vi "PQ_asynchron_sample.vi"() -> ()   [LabVIEW 2019, in "libpqutility64.lvlib"]
doc: "example to show how to communicate asyncronous wir PostgreSQL"
uses:
  libpqutility64.lvlib
  libpqlv64/src/PQgetvalue.vi
  libpqlv64/src/PQnfields.vi
  libpqlv/libpqlv.lvlib
panel:
  out "parameterstatus":string
  out "PQbinaryTuples":i32
  out "PQprotocolVersion":u32
  out "PQnTuples":i32
  out "PQsendQuery":i32
  out "PQerrorMessage":string
  out "PQresultErrorMessage":string
  in  "query":string
  out "PQresultStatus":T1(ring)
  out "PQStatus":T2(ring)
  out "Tabelle":string[][](table)
  in  "conninfo":string
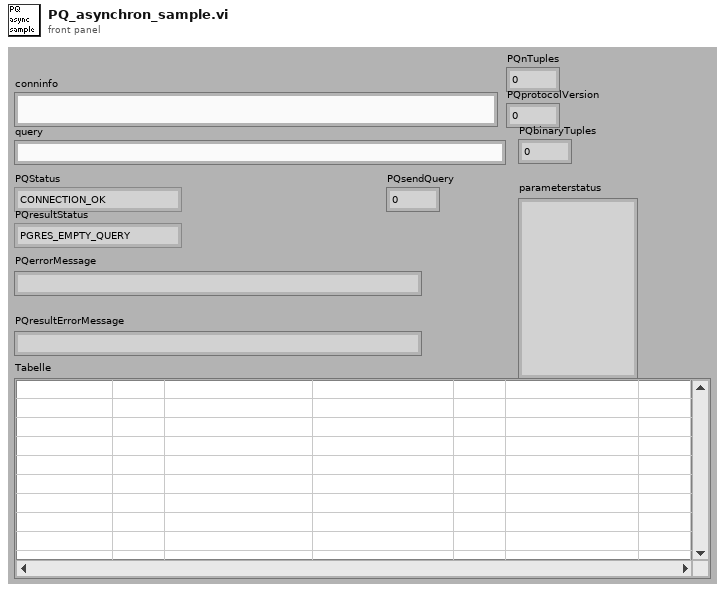
[diagram p1: front panel]
types:
  T1 = enum16{"PGRES_EMPTY_QUERY", "PGRES_COMMAND_OK", "PGRES_TUPLES_OK", "PGRES_COPY_OUT", "PGRES_COPY_IN", "PGRES_BAD_RESPONSE", "PGRES_NONFATAL_ERROR", "PGRES_FATAL_ERROR"}
  T2 = enum16{"CONNECTION_OK", "CONNECTION_BAD", "CONNECTION_STARTED", "CONNECTION_MADE", "CONNECTION_AWAITING_RESPONSE", "CONNECTION_AUTH_OK", "CONNECTION_SETENV", "CONNECTION_SSL_STARTUP", "CONNECTION_NEEDED"}
  T3 = enum32{"CONNECTION_OK", "CONNECTION_BAD", "CONNECTION_STARTED", "CONNECTION_MADE", "CONNECTION_AWAITING_RESPONSE", "CONNECTION_AUTH_OK", "CONNECTION_SETENV", "CONNECTION_SSL_STARTUP", "CONNECTION_NEEDED"}
  T4 = enum32{"PGRES_EMPTY_QUERY", "PGRES_COMMAND_OK", "PGRES_TUPLES_OK", "PGRES_COPY_OUT", "PGRES_COPY_IN", "PGRES_BAD_RESPONSE", "PGRES_NONFATAL_ERROR", "PGRES_FATAL_ERROR"}
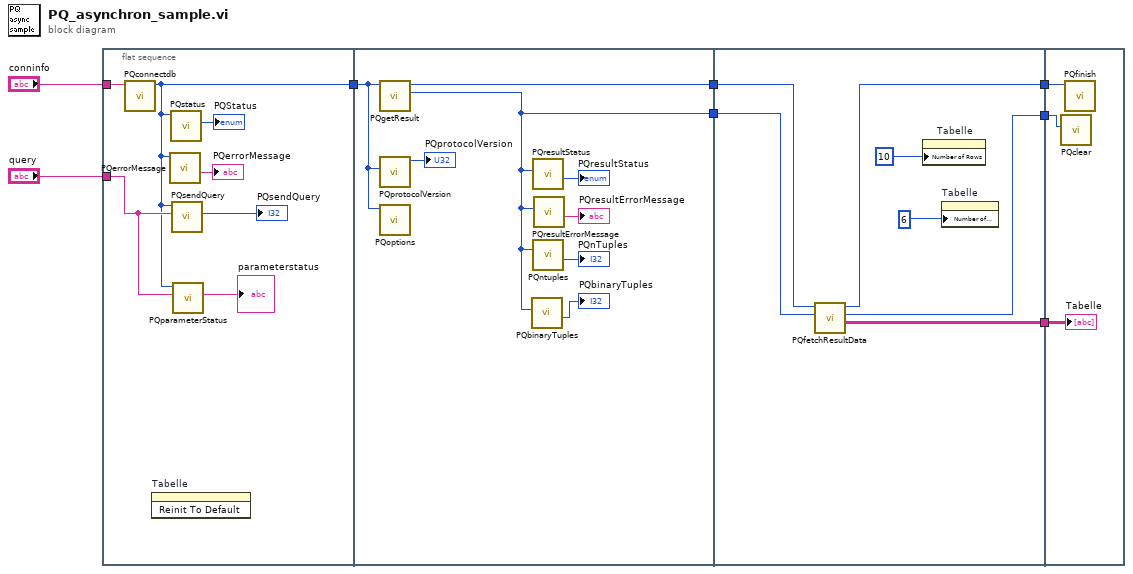
[diagram p0: block diagram]
diagram:
  n1 = flat-sequence {
    tunnel: "conninfo" -> [w15]
    tunnel: "query" -> [w11]
    tunnel: [w10] -> w2
    tunnel: [w17] -> w5
    tunnel: [w21] -> w3
    tunnel: w2 -> [w22]
    tunnel: [w25] -> w6
    tunnel: w5 -> [w24]
    tunnel: [w28] -> w4
    tunnel: w3 -> [w26]
    tunnel: [w27] -> w1
    tunnel: w6 -> [w31]
    tunnel: w4 -> [w33]
    tunnel: w1 -> [w32]
    frame #0 {
      n2 = call "PQconnectdb.vi"("conninfo"=w15) -> ("conn"=w10:u32)  [unwired: 9 in, 1 out]
      n3 = invoke on="Tabelle" class="Tbl (strikt)" method="Reinit To Default"() -> ()  [unwired: 3 in, 3 out]
      n4 = call "PQerrorMessage.vi"("conn"=w10) -> ("PQerrorMessage"=→"PQerrorMessage":string)  [unwired: 8 in, 2 out]
      n5 = call "PQstatus.vi"("conn"=w10) -> ("PQStatus"=→"PQStatus":T3)  [unwired: 8 in, 2 out]
      n6 = call "PQsendQuery.vi"("query"=w11, "conn"=w10) -> ("PQsendQuery"=→"PQsendQuery":i32)  [unwired: 7 in, 2 out]
      n7 = call "PQparameterStatus.vi"("paramName"=w11, "conn"=w10) -> ("parameterstatus"=→"parameterstatus":string)  [unwired: 6 in, 2 out]
    }
    frame #1 {
      n8 = call "PQgetResult.vi"("conn"=w22) -> ("PGresult"=w21:u32, "conn_out"=w17:u32)  [unwired: 8 in, 1 out]
      n9 = call "PQprotocolVersion.vi"("conn"=w22) -> ("PQprotocolVersion"=→"PQprotocolVersion":u32)  [unwired: 9 in, 1 out]
      n10 = call "PQoptions.vi"("conn"=w22) -> ()  [unwired: 7 in, 3 out]
      n11 = call "PQbinaryTuples.vi"("res"=w21) -> ("PQbinaryTuples"=→"PQbinaryTuples":i32)  [unwired: 8 in, 2 out]
      n12 = call "PQresultStatus.vi"("res"=w21) -> ("PQresultStatus"=→"PQresultStatus":T4)  [unwired: 8 in, 2 out]
      n13 = call "PQntuples.vi"("res"=w21) -> ("PQnTuples"=→"PQnTuples":i32)  [unwired: 8 in, 2 out]
      n14 = call "PQresultErrorMessage.vi"("res"=w21) -> ("PQresultErrorMessage"=→"PQresultErrorMessage":string)  [unwired: 8 in, 2 out]
    }
    frame #2 {
      n15 = call "PQfetchResultData.vi"("res"=w26, "conn"=w24) -> ("Data"=w27:string[][], "res_out"=w28:u64, "conn_out"=w25:u64)  [unwired: 4 in, 3 out]
      n16 = property on="Tabelle" class="Tbl (strict)"("Number of Rows"=u32 10 ("Zeilenanzahl")) -> ()  [unwired: 2 in, 2 out]
      n17 = property on="Tabelle" class="Tbl (strict)"("Number of Columns"=u32 6 ("Spaltenanzahl")) -> ()  [unwired: 2 in, 2 out]
    }
    frame #3 {
      n18 = call "PQclear.vi"("res"=w33) -> ()  [unwired: 9 in, 2 out]
      n19 = call "PQfinish.vi"("conn"=w31) -> ()  [unwired: 10 in, 1 out]
      "Tabelle" <- w32
    }
  }
